vi "PCAP to LV Timestamp.vi"(11 "timestamp_seconds":dbl) -> (3 "LabVIEW Time Stamp":timestamp)   [LabVIEW 2025, in "Automotive Ethernet Bus Monitor UI.lvlib" / "lvwpcap.lvlib"]
uses:
  lvwpcap.lvlib
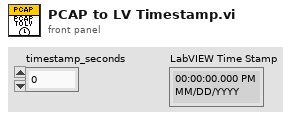
[diagram p1: front panel]
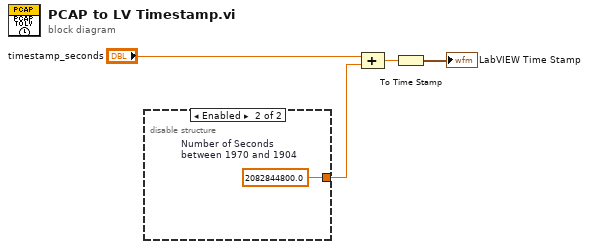
[diagram p0: block diagram]
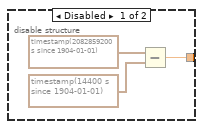
[diagram p2: hidden frame]
diagram:
  n1 = disable-structure "Diagram Disable Structure" shown="Enabled" {
    disable-tunnel: [w5 w8] -> w2
    frame Disabled {
      n2 = Subtract(x=timestamp(2082859200 s since 1904-01-01), y=timestamp(14400 s since 1904-01-01)) -> (x-y=w5:dbl)
    }
    frame Enabled {
      w8 = 2082844800.0  # Number of Seconds between 1970 and 1904
    }
  }
  n3 = Compound Arithmetic op=ADD("timestamp_seconds", w2) -> (w3:dbl)
  n4 = To Time Stamp(1:w3) -> (0:→"LabVIEW Time Stamp":timestamp)
